vi "c ctre phoenixpro encode device.vi"(7 "deviceEncoding":u32, 8 "error in (no error)":errorcluster, 9 "model":string, 10 "deviceId":i32, 11 "context":u32(ring) items=["ContextAPI", "ContextDiagServer"]) -> (0 "error out":errorcluster, 3 "function return":i32, 5 "deviceEncoding out":u32)   [LabVIEW 2020, in "CTRE_PhoenixTools.lvlib"]
doc: "CTREXPORT int c_ctre_phoenixpro_encode_device(Context context, int deviceId, const char *model, uint32_t *deviceEncoding);"
uses:
  CTRE_PhoenixTools.lvlib
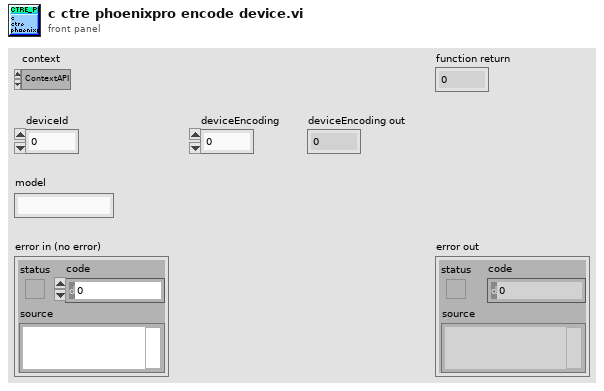
[diagram p1: front panel]
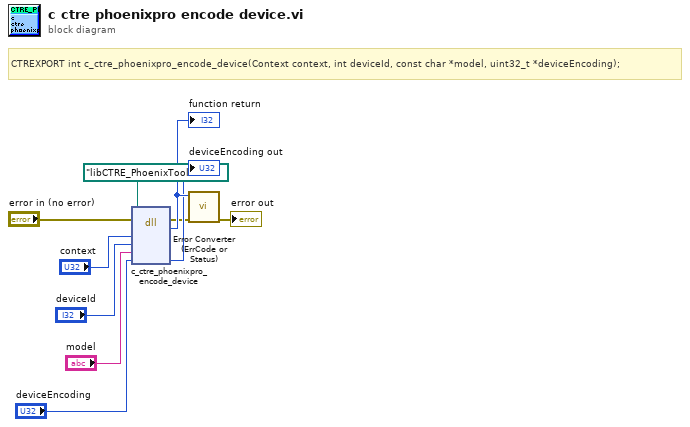
[diagram p0: block diagram]
diagram:
  # "CTREXPORT int c_ctre_phoenixpro_encode_device(Context context, int deviceId, const char *model, uint32_t *deviceEncoding);"
  n1 = dll-call lib="?" fn="c_ctre_phoenixpro_encode_device"(path in=path "libCTRE_PhoenixTools.so", error in="error in (no error)", "context"="context", "deviceId"="deviceId", "model"="model", "deviceEncoding"="deviceEncoding") -> (error out=w3:errorcluster, "return type"=w10:i32, "deviceEncoding"=→"deviceEncoding out":u32)  [unwired: 4 in, 1 out]
  "function return" <- w10
  n2 = call "Error Converter (ErrCode or Status).vi"("error in (no error)"=w3, "error code"=w10) -> ("error out"=→"error out":errorcluster)  [unwired: 9 in]
